vi "onCreate.vi"(8 "error in (no error)":errorcluster, 11 "Client in":refnum<class "Client.lvclass">) -> (0 "error out":errorcluster, 3 "Client out":refnum<class "Client.lvclass">)   [LabVIEW 2013, in "MQTT Client.lvlib" / "Client.lvclass"]
uses:
  Client.lvclass
  Session.Client/Session.Client.lvclass
  Client.lvclass/Client.ctl
  <vilib>/LabVIEW Open Source Project/MQTT Connection/MQTT_Base/Base Class/MQTT_Base.lvclass
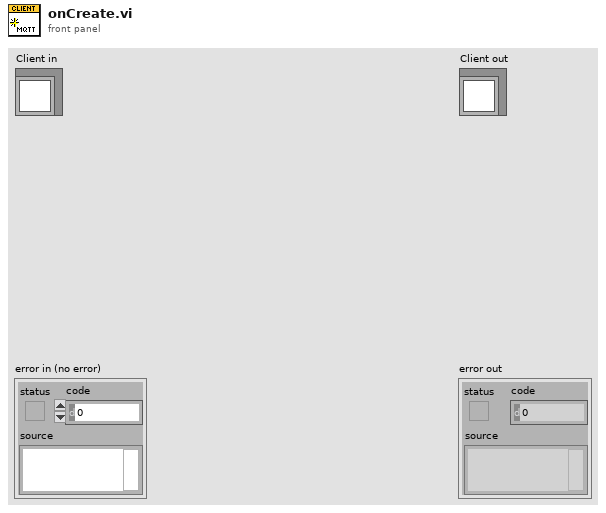
[diagram p1: front panel]
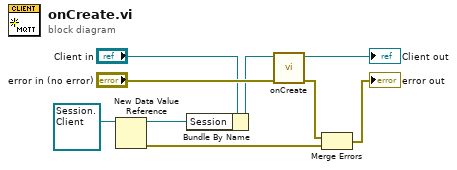
[diagram p0: block diagram]
diagram:
  n1 = New Data Value Reference(data value=refnum<class "Session.Client.lvclass"> refnum ("Session")) -> (data value reference=w6:refnum<data-value>, error out=w3:errorcluster)  [unwired: 1 in]
  n2 = Bundle By Name(cluster="Client in", "Session"=w6) -> (w4:refnum<class "Client.lvclass">)
  n3 = call-parent "onCreate.vi"("error in (no error)"="error in (no error)", "MQTT_Base in"=w4) -> ("error out"=w2:errorcluster, "MQTT_Base out"=→"Client out":refnum<class "Client.lvclass">)  [unwired: 8 in]
  n4 = Merge Errors(w2, w3) -> (→"error out":errorcluster)
